vi "Write Page Runtime Menu Properties.vi"(8 "Error In":errorcluster, 10 "RunTime Menus Properties":T1[](array[typedef]), 11 "Custom Device Page .NET Ref In":refnum<k24>) -> (0 "Error Out":errorcluster, 3 "Custom Device Page .NET Ref Out":refnum<k24>)   [LabVIEW 2019, in "VeriStand Custom Device XML Parser.lvlib"]
doc: "Sets the properties of each runtime menu and sets the array of menu items to the page"
uses:
  VeriStand Custom Device XML Parser.lvlib
  NationalInstruments.VeriStand.XMLReader
  XML Controls/RunTimeMenus Properties.ctl
  XML Controls/Execution Types.ctl
  XML Controls/Path Cluster.ctl
  XML Controls/Dependency Properties.ctl
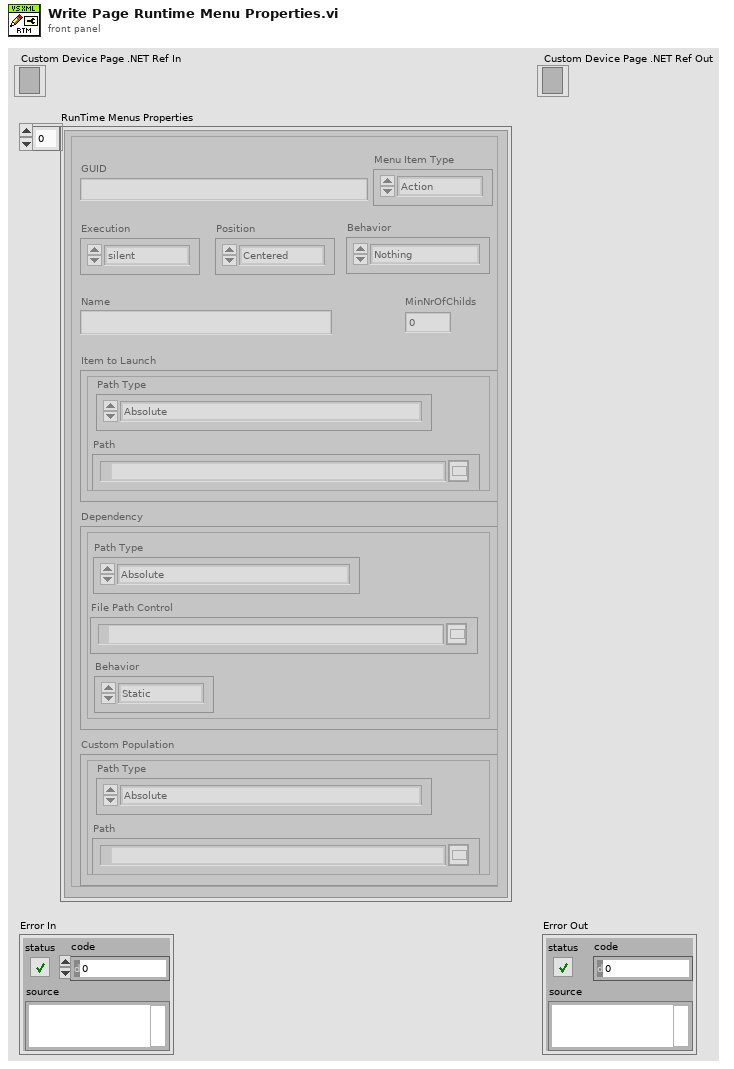
[diagram p1: front panel]
types:
  T1 = typedef "VeriStand Custom Device XML Parser.lvlib/RunTimeMenus Properties.ctl" = cluster{"GUID":string, "Execution":T2, "MinNrOfChilds":u32, "Name":string, "Item to Launch":T3, "Dependency":T4, "Custom Population":T3, "Menu Item Type":enum16{"Action", "VI", "Separator", "Custom"}, "Behavior":enum16{"Nothing", "Open Front Panel"}, "Position":enum16{"Centered", "Mouse Pointer"}}
  T2 = typedef "VeriStand Custom Device XML Parser.lvlib/Execution Types.ctl" = enum16{"silent", "modal", "floating", "default"}
  T3 = typedef "VeriStand Custom Device XML Parser.lvlib/Path Cluster.ctl" = cluster{"Path":path, "Path Type":enum16{"Absolute", "To Base", "To Common Doc Dir", "To Application Data Dir"}}
  T4 = typedef "VeriStand Custom Device XML Parser.lvlib/Dependency Properties.ctl" = cluster{"File Path Control":path, "Path Type":enum16{"Absolute", "To Base", "To Common Doc Dir", "To Application Data Dir"}, "Behavior":enum16{"Static", "Dynamic"}}
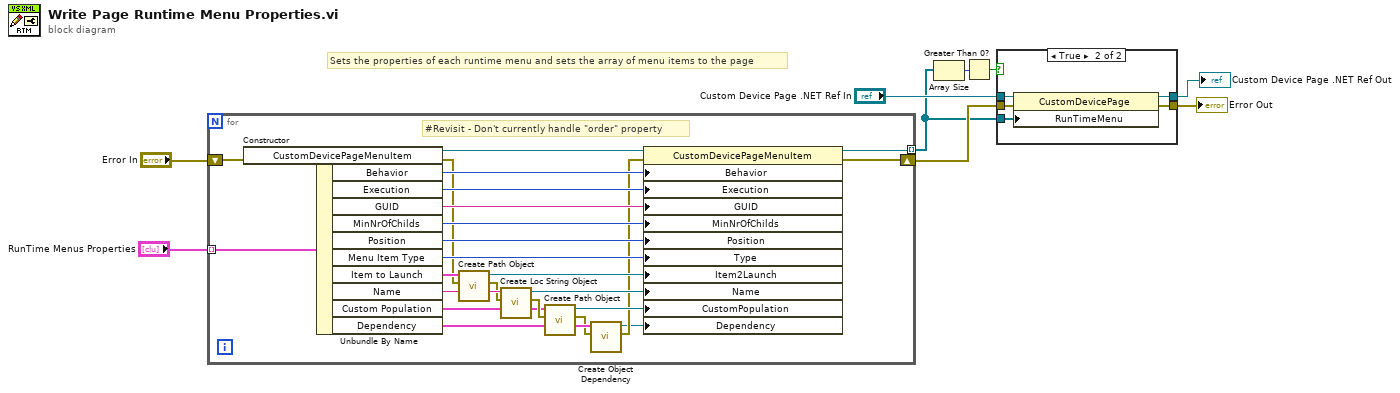
[diagram p0: block diagram]
diagram:
  # "Sets the properties of each runtime menu and sets the array of menu items to the page"
  n1 = for {
    tunnel: "RunTime Menus Properties" -> [w33] mode=indexing
    shift-right: [w15] -> w7
    shift-left: "Error In" -> [w32]
    tunnel: [w14] -> w1 mode=indexing
    # "#Revisit - Don't currently handle \"order\" property"
    n2 = constructor class="CustomDevicePageMenuItem"(error in=w32) -> (reference out=w31:refnum<k24>, error out=w23:errorcluster)  [unwired: 2 in, 1 out]
    n3 = Unbundle By Name(w33) -> ("Behavior"=w30:enum16{"Nothing", "Open Front Panel"}, "Execution"=w29:T2, "GUID"=w28:string, "MinNrOfChilds"=w27:u32, "Position"=w26:enum16{"Centered", "Mouse Pointer"}, "Menu Item Type"=w25:enum16{"Action", "VI", "Separator", "Custom"}, "Item to Launch"=w24:T3, "Name"=w21:string, "Custom Population"=w17:T3, "Dependency"=w13:T4)
    n4 = call "Create Path Object.vi"("Error In"=w23, "Path Data Cluster"=w24) -> ("Error Out"=w20:errorcluster, "Path .NET Ref"=w22:refnum<k24>)  [unwired: 8 in]
    n5 = call "Create Loc String Object.vi"("Error In"=w20, "String Input"=w21) -> ("Error Out"=w18:errorcluster, "Loc String .NET Ref"=w19:refnum<k24>)  [unwired: 8 in]
    n6 = call "Create Path Object.vi"("Error In"=w18, "Path Data Cluster"=w17) -> ("Error Out"=w12:errorcluster, "Path .NET Ref"=w16:refnum<k24>)  [unwired: 8 in]
    n7 = call "Create Object Dependency.vi"("Error In"=w12, "Dependency Properties"=w13) -> ("Error Out"=w11:errorcluster, "Dependency .NET Ref Out"=w10:refnum<k24>)  [unwired: 8 in]
    n8 = property class="CustomDevicePageMenuItem"(reference=w31, error in=w11, "Behavior"=w30, "Execution"=w29, "GUID"=w28, "MinNrOfChilds"=w27, "Position"=w26, "Type"=w25, "Item2Launch"=w22, "Name"=w19, "CustomPopulation"=w16, "Dependency"=w10) -> (reference out=w14:refnum<k24>, error out=w15:errorcluster)
  }
  n9 = Array Size(array=w1) -> (size(s)=w2:i32)
  n10 = Greater Than 0?(x=w2) -> (x > 0?=w3:bool)
  n11 = case shown="True" w3 {
    tunnel: [w34 w40] -> w9
    tunnel: [w35 w39] -> w8
    tunnel: w1 -> [_ w38]
    tunnel: w7 -> [w34 w37]
    tunnel: "Custom Device Page .NET Ref In" -> [w35 w36]
    frame False {
    }
    frame True {
      n12 = property class="CustomDevicePage"(reference=w36, error in=w37, "RunTimeMenu"=w38) -> (reference out=w39:refnum<k24>, error out=w40:errorcluster)
    }
  }
  "Error Out" <- w9
  "Custom Device Page .NET Ref Out" <- w8
